vi "XY Graph Get Plot Metadata Type.vi"(8 "Error In":errorcluster, 11 "Graph Label":string) -> (0 "Error Out":errorcluster, 1 "Found?":bool, 3 "Plot Metadata Type":variant)   [LabVIEW 2021, in "XY Graph Add-Ons.lvlib"]
uses:
  XY Graph Add-Ons.lvlib
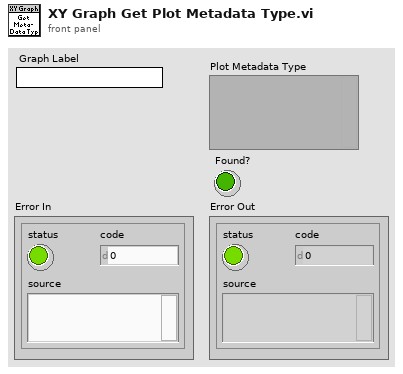
[diagram p1: front panel]
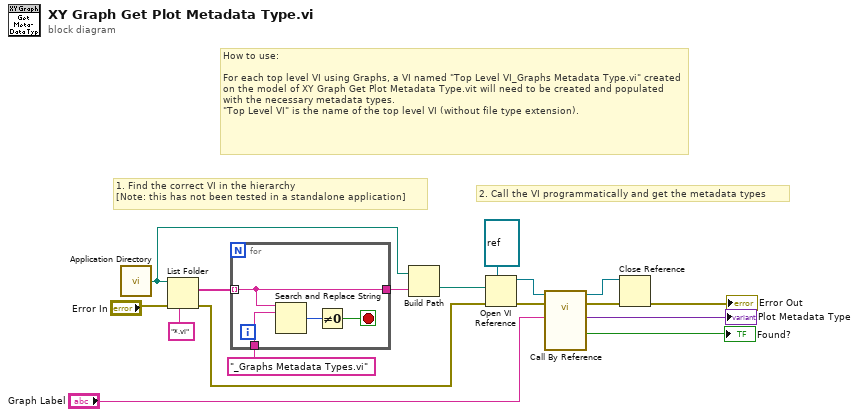
[diagram p0: block diagram]
diagram:
  # "2. Call the VI programmatically and get the metadata types"
  # "1. Find the correct VI in the hierarchy\n[Note: this has not been tested in a standalone application]"
  # "How to use:\n\nFor each top level VI using Graphs, a VI named \"Top Level VI_Graphs Metadata Type.vi\" created on the model of XY Graph Get Plot Metadata Type.vit will need to be created and populated with the necessary metadata types.\n\"Top Level VI\" is the name of the top level VI (without file type extension)."
  n1 = call <vilib>:"Application Directory.vi"() -> ("Application Directory"=w3:path)
  n2 = List Folder(path=w3, pattern="*.vi", error in="Error In") -> (filenames=w6:string[], error out=w1:errorcluster)  [unwired: 1 in, 2 out]
  n3 = for {
    tunnel: w6 -> [w18] mode=indexing
    tunnel: "_Graphs Metadata Types.vi" ("string") -> [w21]
    tunnel: [w18] -> w4
    stop <- w19 stop-if-true
    n4 = Search and Replace String(input string=w18, search string=w21) -> (number of replacements=w20:i32)  [unwired: 6 in, 3 out]
    n5 = Not Equal To 0?(x=w20) -> (x != 0?=w19:bool)
  }
  n6 = Build Path(base path=w3, name or relative path=w4) -> (appended path=w2:path)
  n7 = Open VI Reference(type specifier VI Refnum (for type only)=refnum<vi> refnum, vi path=w2, error in (no error)=w1) -> (vi reference=w13:refnum<vi>, error out=w14:errorcluster)  [unwired: 3 in]
  n8 = call-by-ref "?"(reference=w13, error in=w14, "Graph Label"="Graph Label") -> (reference out=w11:refnum<vi>, error out=w10:errorcluster, "Found?"=→"Found?":bool, "Plot Metadata Type"=→"Plot Metadata Type":variant)  [unwired: 9 in]
  n9 = Close Reference(reference=w11, error in (no error)=w10) -> (error out=→"Error Out":errorcluster)
